vi "Msg To.vi"(10 "Event jettl":refnum<class "Event jettl.lvclass">) -> (3 "Event Last Ack Msg Strategy out":refnum<class "Event Last Ack Msg Strategy.lvclass">)   [LabVIEW 2021, in "jettl.lvlib" / "Event Last Ack.lvlib"]
uses:
  Event Last Ack.lvlib
  Event jettl/Event jettl.lvclass
  Event Last Ack Msg Strategy/Event Last Ack Msg Strategy.lvclass
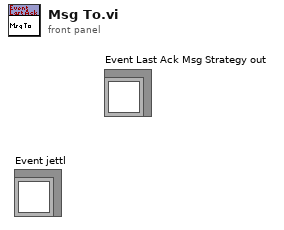
[diagram p1: front panel]
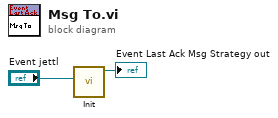
[diagram p0: block diagram]
diagram:
  n1 = call "Init.vi"("Event jettl"="Event jettl") -> ("Event Last Ack Msg Strategy out"=→"Event Last Ack Msg Strategy out":refnum<class "Event Last Ack Msg Strategy.lvclass">)  [unwired: 10 in]
